vi "create_position_file_paths.vi"(5 "number of position channels":i32=3, 7 "index of first position channel":i32=2, 8 "error in (no error)":errorcluster, 10 "image file path":path) -> (0 "error out":errorcluster, 2 "x/y/z path":path[](array[path]))   [LabVIEW 2010, in "PositionSignals.lvclass"]
uses:
  PositionSignals.lvclass
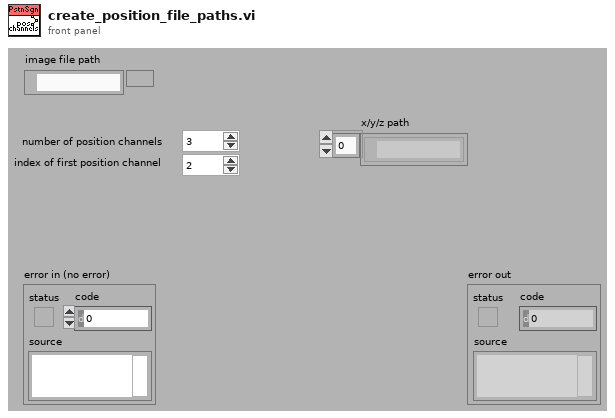
[diagram p1: front panel]
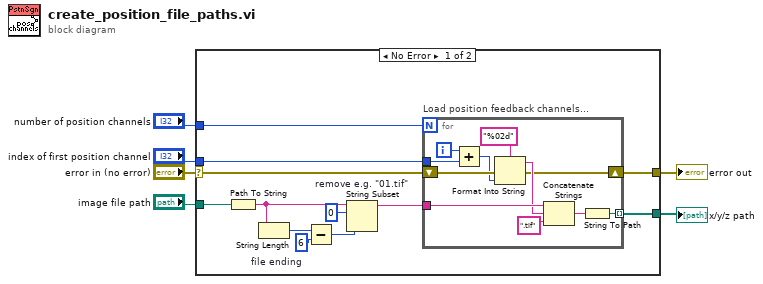
[diagram p0: block diagram]
diagram:
  n1 = case shown="No Error" "error in (no error)" {
    selector: "error in (no error)" -> [w12 w30]
    tunnel: [w11 w30] -> w5
    tunnel: "image file path" -> [w13 _]
    tunnel: "index of first position channel" -> [w9 _]
    tunnel: "number of position channels" -> [w8 _]
    tunnel: [w7 _] -> w1
    frame No Error {
      w17 = 6  # file ending
      n2 = Path To String(path=w13) -> (string=w15:string)
      n3 = String Length(string=w15) -> (length=w16:i32)
      n4 = Subtract(x=w16, y=w17) -> (x-y=w18:i32)
      n5 = String Subset "remove e.g. \"01.tif\""(string=w15, offset (0)=0, length (rest)=w18) -> (substring=w10:string)
      n6 = for "Load position feedback channels..." {
        N: w8 -> [_]
        shift-right: [w20] -> w11
        shift-left: w12 -> [w26]
        tunnel: w10 -> [w25]
        tunnel: w9 -> [w21]
        tunnel: [w19] -> w7 mode=indexing
        i -> [w27]
        n7 = Add(x=w27, y=w21) -> (x+y=w22:i32)
        n8 = Format Into String(format string="%02d", error in=w26, w22) -> (resulting string=w24:string, error out=w20:errorcluster)  [unwired: 1 in]
        n9 = Concatenate Strings(w25, w24, ".tif" ("string")) -> (w29:string)
        n10 = String To Path(string=w29) -> (path=w19:path)
      }
    }
    frame Error {
    }
  }
  "error out" <- w5
  "x/y/z path" <- w1
